vi "2d to boolean sub vi.vi"(11 "Numeric":dbl) -> (3 "initialized array":bool[][](array[boolean]))   [LabVIEW 2020]
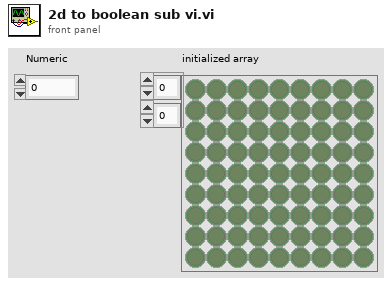
[diagram p1: front panel]
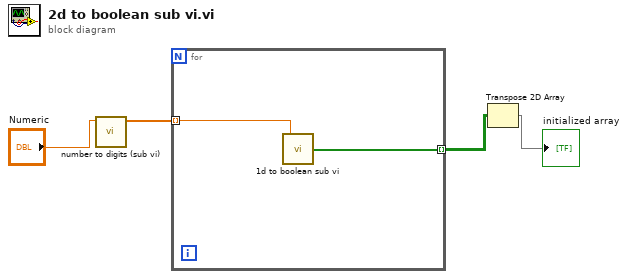
[diagram p0: block diagram]
diagram:
  n1 = call "number to digits (sub vi).vi"("Numeric"="Numeric") -> ("reversed array"=w2:dbl[])  [unwired: 10 in]
  n2 = for {
    tunnel: w2 -> [w6] mode=indexing
    tunnel: [w5] -> w3 mode=indexing
    n3 = call "1d to boolean sub vi.vi"("A"=w6) -> ("initialized array"=w5:bool[])
  }
  n4 = Transpose 2D Array(2D array=w3) -> (transposed array=→"initialized array":bool[][])
